vi "binaryarray2integer.vi"(11 "Array":dbl[](array[numeric])) -> (0 "Answer":dbl)   [LabVIEW 2016]
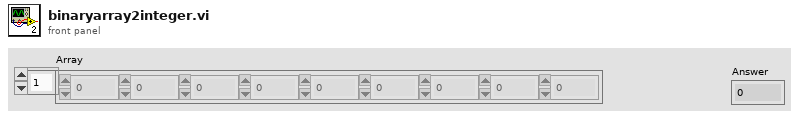
[diagram p1: front panel]
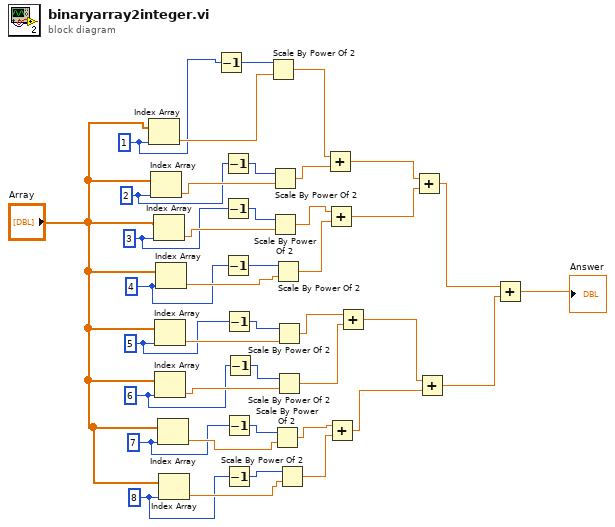
[diagram p0: block diagram]
diagram:
  w14 = 8
  w12 = 7
  w10 = 6
  w8 = 5
  w6 = 4
  w4 = 3
  w3 = 2
  w16 = 1
  n1 = Index Array(array="Array", index=w16) -> (element=w31:dbl)
  n2 = Index Array(array="Array", index=w3) -> (element=w17:dbl)
  n3 = Index Array(array="Array", index=w4) -> (element=w23:dbl)
  n4 = Index Array(array="Array", index=w8) -> (element=w21:dbl)
  n5 = Index Array(array="Array", index=w10) -> (element=w20:dbl)
  n6 = Index Array(array="Array", index=w6) -> (element=w22:dbl)
  n7 = Index Array(array="Array", index=w12) -> (element=w19:dbl)
  n8 = Index Array(array="Array", index=w14) -> (element=w18:dbl)
  n9 = Decrement(x=w16) -> (x-1=w15:i32)
  n10 = Decrement(x=w3) -> (x-1=w2:i32)
  n11 = Decrement(x=w4) -> (x-1=w1:i32)
  n12 = Decrement(x=w6) -> (x-1=w5:i32)
  n13 = Decrement(x=w8) -> (x-1=w7:i32)
  n14 = Decrement(x=w12) -> (x-1=w11:i32)
  n15 = Decrement(x=w14) -> (x-1=w13:i32)
  n16 = Decrement(x=w10) -> (x-1=w9:i32)
  n17 = Scale By Power Of 2(n=w15, x=w31) -> (x*2^n=w32:dbl)
  n18 = Scale By Power Of 2(n=w2, x=w17) -> (x*2^n=w26:dbl)
  n19 = Scale By Power Of 2(n=w1, x=w23) -> (x*2^n=w25:dbl)
  n20 = Scale By Power Of 2(n=w11, x=w19) -> (x*2^n=w29:dbl)
  n21 = Scale By Power Of 2(n=w5, x=w22) -> (x*2^n=w24:dbl)
  n22 = Scale By Power Of 2(n=w7, x=w21) -> (x*2^n=w27:dbl)
  n23 = Scale By Power Of 2(n=w9, x=w20) -> (x*2^n=w28:dbl)
  n24 = Scale By Power Of 2(n=w13, x=w18) -> (x*2^n=w30:dbl)
  n25 = Add(x=w32, y=w26) -> (x+y=w33:dbl)
  n26 = Add(x=w25, y=w24) -> (x+y=w34:dbl)
  n27 = Add(x=w29, y=w30) -> (x+y=w35:dbl)
  n28 = Add(x=w27, y=w28) -> (x+y=w36:dbl)
  n29 = Add(x=w33, y=w34) -> (x+y=w37:dbl)
  n30 = Add(x=w36, y=w35) -> (x+y=w38:dbl)
  n31 = Add(x=w37, y=w38) -> (x+y=→"Answer":dbl)
